vi "NHMFL Visible Optics.vi"() -> ()   [LabVIEW 2019]
panel:
  in  "Case Constant\n(See Context Help) 2":bool=TRUE
  in  "Case Constant\n(See Context Help)":bool=TRUE
  in  "Loading State":T1(ring)=enum."Load Globals"
  # "Welcome to NHMFL\nVisible Optics Facility\n\n\n(Program Loading...)"
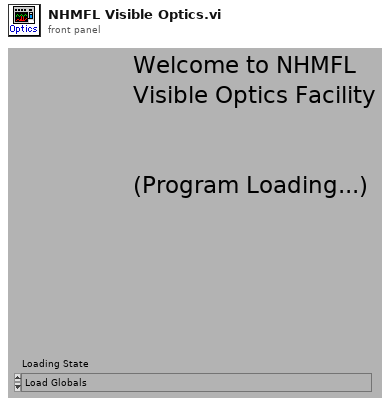
[diagram p1: front panel]
types:
  T1 = enum16{"--Quit--", "Load Globals", "Load Master", "Load Spectrometer", "Load Field", "Load Temperature", "Load Misc"}
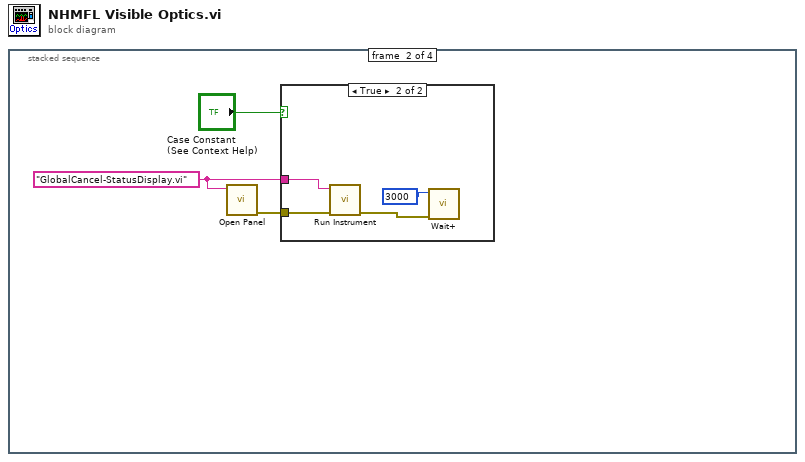
[diagram p0: block diagram]
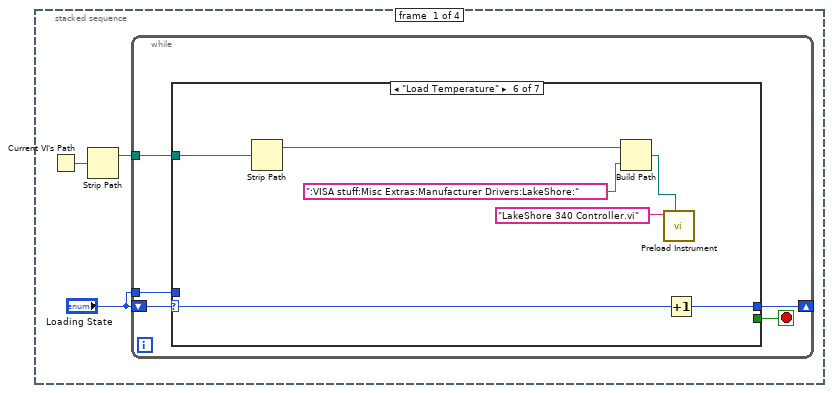
[diagram p2: hidden frame]
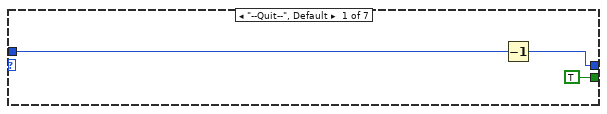
[diagram p3: hidden frame]
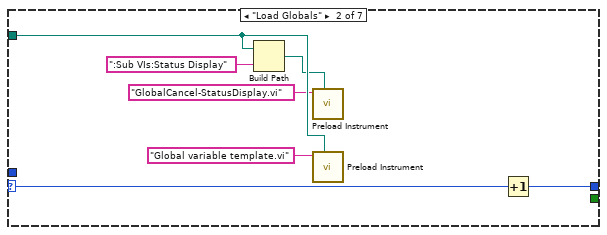
[diagram p4: hidden frame]
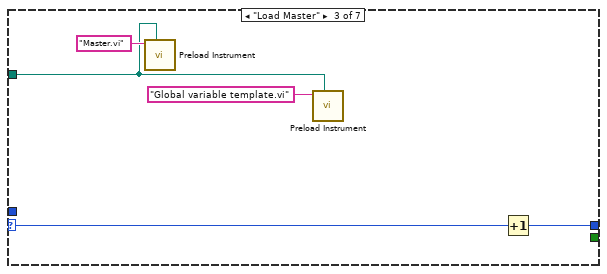
[diagram p5: hidden frame]
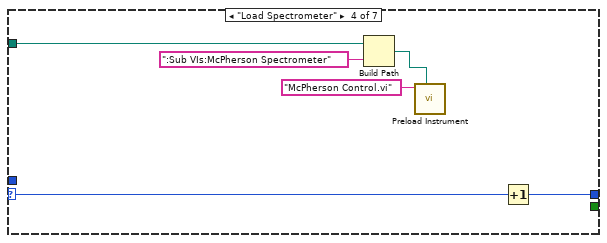
[diagram p6: hidden frame]
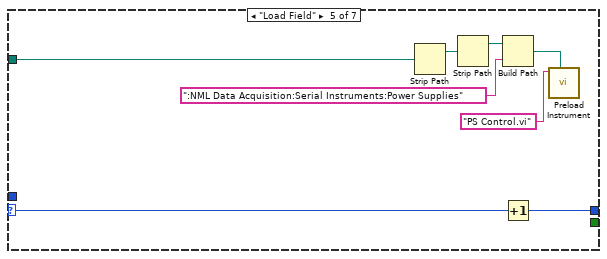
[diagram p7: hidden frame]
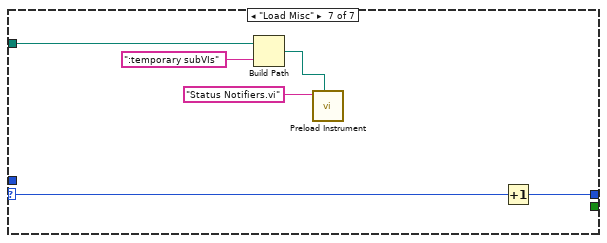
[diagram p8: hidden frame]
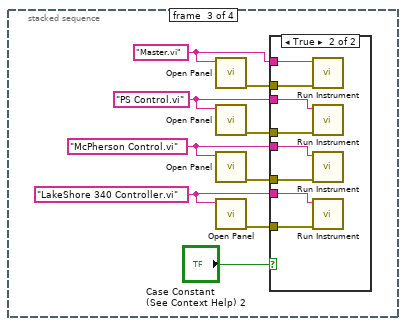
[diagram p10: hidden frame]
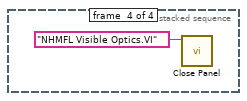
[diagram p12: hidden frame]
diagram:
  n1 = stacked-sequence {
    frame #0 {
      n2 = Current VI's Path() -> (path=w2:path)
      n3 = Strip Path(path=w2) -> (stripped path=w1:path)  [unwired: 1 out]
      n4 = while {
        shift-right: [w7] -> _
        shift-left: "Loading State" -> [w8]
        tunnel: "Loading State" -> [w6]
        tunnel: w1 -> [w5]
        stop <- w4 stop-if-true
        n5 = case shown="\"Load Temperature\"" w8 {
          selector: w8 -> [_ w17 w22 w28 w36 w43 w49]
          tunnel: [w11 w18 w23 w29 w37 w44 w50] -> w7
          tunnel: w6 -> [w10 _ _ _ _ _ _]
          tunnel: w5 -> [_ w15 w19 w26 w31 w39 w47]
          tunnel: [TRUE _ _ _ _ _ _] -> w4
          frame "--Quit--", Default {
            n6 = Decrement(x=w10) -> (x-1=w11:T1)
          }
          frame "Load Globals" {
            n7 = Build Path(base path=w15, name or relative path=":Sub VIs:Status Display") -> (appended path=w13:path)
            n8 = call <vilib>:"Preload Instrument.vi"("VI path"=w13, "VI name"="GlobalCancel-StatusDisplay.vi" ("name or relative path")) -> ()  [unwired: 9 in, 1 out]
            n9 = call <vilib>:"Preload Instrument.vi"("VI path"=w15, "VI name"="Global variable template.vi" ("name or relative path")) -> ()  [unwired: 9 in, 1 out]
            n10 = Increment(x=w17) -> (x+1=w18:T1)
          }
          frame "Load Master" {
            n11 = call <vilib>:"Preload Instrument.vi"("VI path"=w19, "VI name"="Master.vi" ("name or relative path")) -> ()  [unwired: 9 in, 1 out]
            n12 = call <vilib>:"Preload Instrument.vi"("VI path"=w19, "VI name"="Global variable template.vi" ("name or relative path")) -> ()  [unwired: 9 in, 1 out]
            n13 = Increment(x=w22) -> (x+1=w23:T1)
          }
          frame "Load Spectrometer" {
            n14 = Build Path(base path=w26, name or relative path=":Sub VIs:McPherson Spectrometer") -> (appended path=w25:path)
            n15 = call <vilib>:"Preload Instrument.vi"("VI path"=w25, "VI name"="McPherson Control.vi" ("name or relative path")) -> ()  [unwired: 9 in, 1 out]
            n16 = Increment(x=w28) -> (x+1=w29:T1)
          }
          frame "Load Field" {
            n17 = Strip Path(path=w31) -> (stripped path=w32:path)  [unwired: 1 out]
            n18 = Strip Path(path=w32) -> (stripped path=w33:path)  [unwired: 1 out]
            n19 = Build Path(base path=w33, name or relative path=":NML Data Acquisition:Serial Instruments:Power Supplies") -> (appended path=w30:path)
            n20 = Increment(x=w36) -> (x+1=w37:T1)
            n21 = call <vilib>:"Preload Instrument.vi"("VI path"=w30, "VI name"="PS Control.vi" ("name or relative path")) -> ()  [unwired: 9 in, 1 out]
          }
          frame "Load Temperature" {
            n22 = Strip Path(path=w39) -> (stripped path=w38:path)  [unwired: 1 out]
            n23 = Build Path(base path=w38, name or relative path=":VISA stuff:Misc Extras:Manufacturer Drivers:LakeShore:") -> (appended path=w41:path)
            n24 = call <vilib>:"Preload Instrument.vi"("VI path"=w41, "VI name"="LakeShore 340 Controller.vi" ("name or relative path")) -> ()  [unwired: 9 in, 1 out]
            n25 = Increment(x=w43) -> (x+1=w44:T1)
          }
          frame "Load Misc" {
            n26 = Build Path(base path=w47, name or relative path=":temporary subVIs") -> (appended path=w46:path)
            n27 = call <vilib>:"Preload Instrument.vi"("VI path"=w46, "VI name"="Status Notifiers.vi" ("name or relative path")) -> ()  [unwired: 9 in, 1 out]
            n28 = Increment(x=w49) -> (x+1=w50:T1)
          }
        }
      }
    }
    frame #1 {
      w52 = "GlobalCancel-StatusDisplay.vi" ("name or relative path")
      n29 = call <vilib>:"Open Panel.vi"("VI name"=w52) -> ("error out"=w53:errorcluster)  [unwired: 10 in]
      n30 = case shown="True" "Case Constant\n(See Context Help)" {
        tunnel: w53 -> [_ w57]
        tunnel: w52 -> [_ w56]
        frame False {
        }
        frame True {
          n31 = call <vilib>:"Run Instrument.vi"("error in (no error)"=w57, "VI name"=w56) -> ("error out"=w55:errorcluster)  [unwired: 9 in]
          n32 = call "Wait+.vi"("Error In"=w55, "milliseconds to wait"=u32 3000) -> ()  [unwired: 4 in, 2 out]
        }
      }
    }
    frame #2 {
      w58 = "PS Control.vi" ("name or relative path")
      w61 = "LakeShore 340 Controller.vi" ("name or relative path")
      w62 = "Master.vi" ("name or relative path")
      w63 = "McPherson Control.vi" ("name or relative path")
      n33 = call <vilib>:"Open Panel.vi"("VI name"=w62) -> ("error out"=w65:errorcluster)  [unwired: 10 in]
      n34 = call <vilib>:"Open Panel.vi"("VI name"=w58) -> ("error out"=w60:errorcluster)  [unwired: 10 in]
      n35 = call <vilib>:"Open Panel.vi"("VI name"=w63) -> ("error out"=w66:errorcluster)  [unwired: 10 in]
      n36 = call <vilib>:"Open Panel.vi"("VI name"=w61) -> ("error out"=w64:errorcluster)  [unwired: 10 in]
      n37 = case shown="True" "Case Constant\n(See Context Help) 2" {
        tunnel: w66 -> [_ w74]
        tunnel: w65 -> [_ w73]
        tunnel: w64 -> [_ w72]
        tunnel: w63 -> [_ w71]
        tunnel: w62 -> [_ w70]
        tunnel: w61 -> [_ w69]
        tunnel: w60 -> [_ w68]
        tunnel: w58 -> [_ w67]
        frame False {
        }
        frame True {
          n38 = call <vilib>:"Run Instrument.vi"("error in (no error)"=w73, "VI name"=w70) -> ()  [unwired: 9 in, 1 out]
          n39 = call <vilib>:"Run Instrument.vi"("error in (no error)"=w68, "VI name"=w67) -> ()  [unwired: 9 in, 1 out]
          n40 = call <vilib>:"Run Instrument.vi"("error in (no error)"=w74, "VI name"=w71) -> ()  [unwired: 9 in, 1 out]
          n41 = call <vilib>:"Run Instrument.vi"("error in (no error)"=w72, "VI name"=w69) -> ()  [unwired: 9 in, 1 out]
        }
      }
    }
    frame #3 {
      n42 = call <vilib>:"Close Panel.vi"("VI name"="NHMFL Visible Optics.VI") -> ()  [unwired: 10 in, 1 out]
    }
  }
